vi "Read Intternal Pathloss Value.vi"(10 "Center Frequency, Hz":dbl=5185000000.0, 11 "file path":path) -> (3 "External Attenuation, dB":dbl format="%.2f")   [LabVIEW 2012]
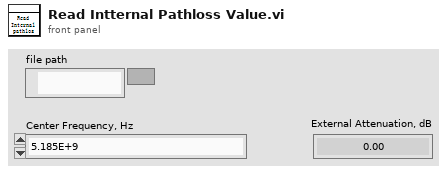
[diagram p1: front panel]
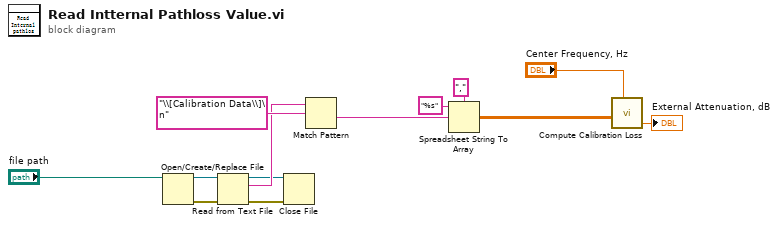
[diagram p0: block diagram]
diagram:
  n1 = Open/Create/Replace File(file path (use dialog)="file path") -> (refnum out=w5:refnum<file>, error out=w6:errorcluster)  [unwired: 5 in, 1 out]
  n2 = Read from Text File(file (use dialog)=w5, error in=w6) -> (refnum out=w7:refnum<file>, text=w9:string, error out=w8:errorcluster)  [unwired: 2 in, 1 out]
  n3 = Close File(refnum=w7, error in=w8) -> ()  [unwired: 2 out]
  n4 = Match Pattern(string=w9, regular expression="\\[Calibration Data\\]\n") -> (after substring=w11:string)  [unwired: 1 in, 3 out]
  n5 = Spreadsheet String To Array(delimiter (Tab)=",", format string="%s", spreadsheet string=w11) -> (array=w4:dbl[][])  [unwired: 1 in]
  n6 = call "Compute Calibration Loss.vi"("Table (frequency, power, pathloss)"=w4, "Center Frequency, Hz"="Center Frequency, Hz") -> ("External Attenuation, dB"=→"External Attenuation, dB":dbl)  [unwired: 3 in, 2 out]
